vi "Init Msg.vi"(6 "Teller":refnum<class "Teller.lvclass">) -> (2 "Msg":refnum<class "Msg.lvclass">)   [LabVIEW 2025, in "_Template.lvlib" / "Templates.lvlib" / "TEMPLATE jettl Msg.lvlib" / "TEMPLATE.lvlib"]
uses:
  TEMPLATE.lvlib
  jettl/jettl/Teller/Teller.lvclass
  jettl/jettl/Msg/Msg.lvclass
  TEMPLATE Msg Input/TEMPLATE Msg Input.lvlib
  TEMPLATE Msg/TEMPLATE Msg.lvlib
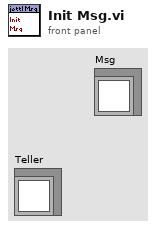
[diagram p1: front panel]
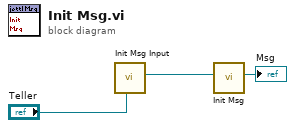
[diagram p0: block diagram]
diagram:
  n1 = call "Init Msg Input.vi"("Teller"="Teller") -> ("Msg Input"=w3:refnum<class "Msg Input.lvclass">)  [unwired: 10 in]
  n2 = call "Init Msg.vi"("Msg Input"=w3) -> ("Msg"=→"Msg":refnum<class "Msg.lvclass">)  [unwired: 10 in]
